vi "DOE Dryer EF Standby Power.vi"(6 "Appliance Common":T1, 8 "Error In":errorcluster, 11 "Standby Power In":T2={"Standby Power Spreadsheet"=[], "Standby Power - Pia (Watts)"=0.0, "Off Mode Power - Poff (Watts)"=0.0, "Sia hr/yr"=8620.0, "Soff hr/yr"=0.0, "Yearly Energy Etso kWh/yr"=0.0, "Maximum Power (Watts)"=0.0, "Power Variation (%)"=0.0, "Slope (mW/hr)"=0.0, "Final Harmonics-U1 (%)"="", "Final Harmonics-U2 (%)"="", "Energy (Wh)"=0.0}) -> (0 "Error Out":errorcluster, 3 "Standby Power Out":T2={"Standby Power Spreadsheet"=[], "Standby Power - Pia (Watts)"=0.0, "Off Mode Power - Poff (Watts)"=0.0, "Sia hr/yr"=8620.0, "Soff hr/yr"=0.0, "Yearly Energy Etso kWh/yr"=0.0, "Maximum Power (Watts)"=0.0, "Power Variation (%)"=0.0, "Slope (mW/hr)"=0.0, "Final Harmonics-U1 (%)"="", "Final Harmonics-U2 (%)"="", "Energy (Wh)"=0.0})   [LabVIEW 2018]
uses:
  Utility/Standby Power/Type Definitions/Standby Power Main Data.ctl
  Type Definitions/DOE Appliance Common.ctl
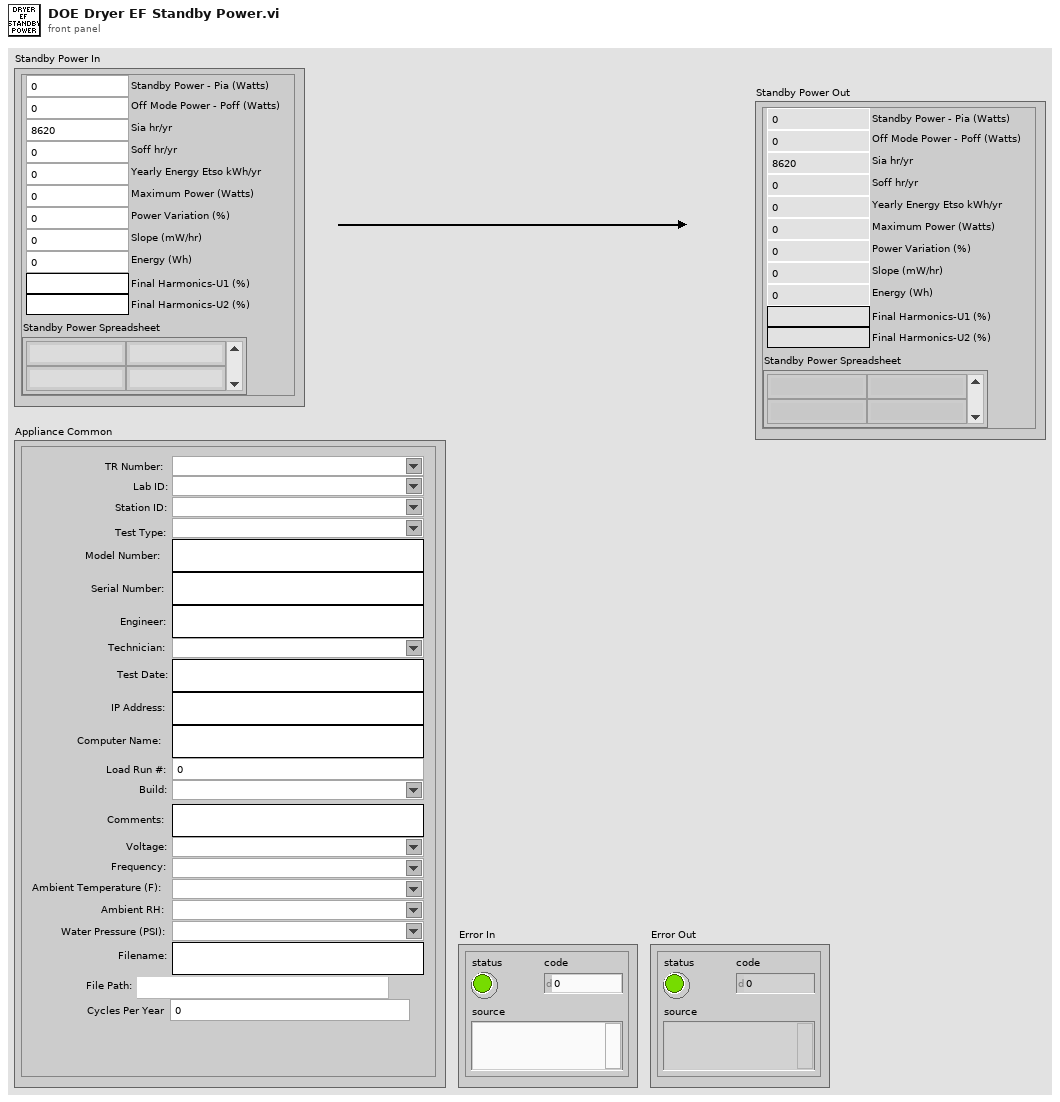
[diagram p1: front panel]
types:
  T1 = typedef "DOE Appliance Common.ctl" = cluster{"Engineer:":string, "Model Number:":string, "Serial Number:":string, "Comments:":string, "Station ID:":string, "Technician:":string, "TR Number:":string, "Lab ID:":string, "Voltage:":string, "Water Pressure (PSI):":string, "Test Date:":string, "Computer Name:":string, "IP Address:":string, "Ambient RH:":string, "Frequency:":string, "Build:":string, "Filename:":string, "Test Type:":string, "Load Run #:":i32, "Ambient Temperature (F):":string, "File Path:":path, "Cycles Per Year":u32}
  T2 = typedef "Standby Power Main Data.ctl" = cluster{"Standby Power Spreadsheet":string[][], "Standby Power - Pia (Watts)":dbl, "Off Mode Power - Poff (Watts)":dbl, "Sia hr/yr":dbl, "Soff hr/yr":dbl, "Yearly Energy Etso kWh/yr":dbl, "Maximum Power (Watts)":dbl, "Power Variation (%)":dbl, "Slope (mW/hr)":dbl, "Final Harmonics-U1 (%)":string, "Final Harmonics-U2 (%)":string, "Energy (Wh)":dbl}
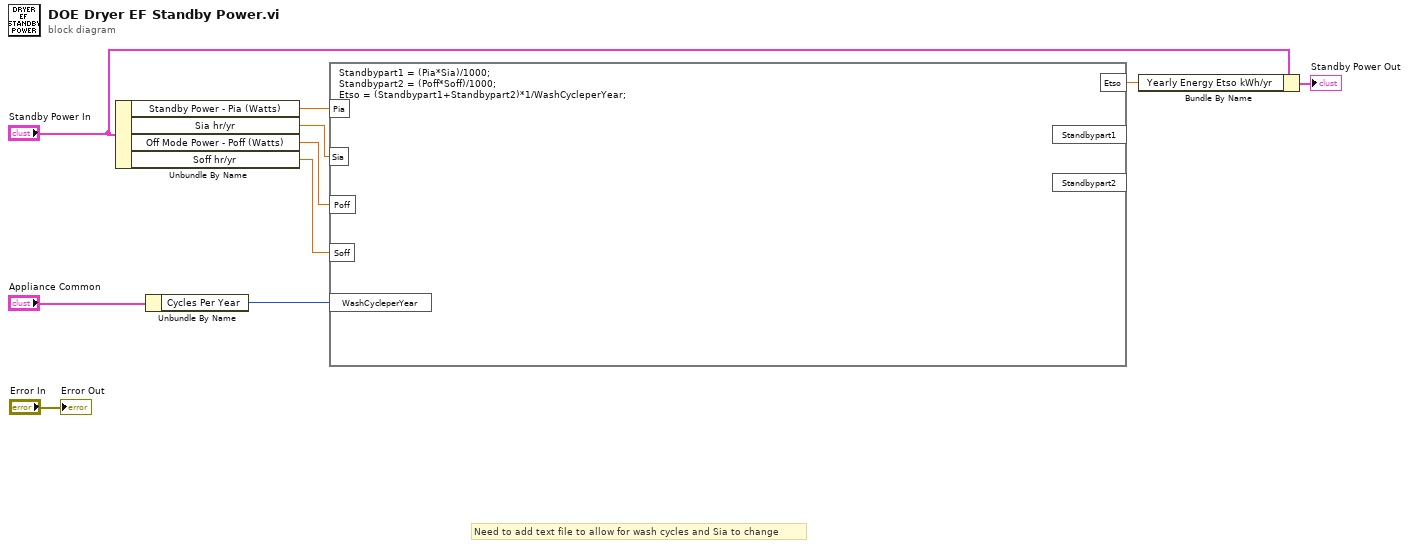
[diagram p0: block diagram]
diagram:
  # "Need to add text file to allow for wash cycles and Sia to change"
  n1 = Unbundle By Name("Standby Power In") -> ("Standby Power - Pia (Watts)"=w9:dbl, "Sia hr/yr"=w8:dbl, "Off Mode Power - Poff (Watts)"=w7:dbl, "Soff hr/yr"=w6:dbl)
  n2 = Unbundle By Name("Appliance Common") -> ("Cycles Per Year"=w1:u32)
  n3 = formula code="Standbypart1 = (Pia*Sia)/1000;\nStandbypart2 = (Poff*Soff)/1000;\nEtso = (Standbypart1+Standbypart2)*1/WashCycleperYear;"("Pia"=w9, "Sia"=w8, "Poff"=w7, "Soff"=w6, "WashCycleperYear"=w1) -> ("Etso"=w4:dbl)  [unwired: 2 out]
  n4 = Bundle By Name(cluster="Standby Power In", "Yearly Energy Etso kWh/yr"=w4) -> (→"Standby Power Out":T2)
  "Error Out" <- "Error In"
